vi "FilmVariable.vi"() -> ()   [LabVIEW 2015]
panel:
  out "Film Height":dbl
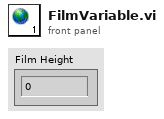
[diagram p1: front panel]
diagram:
